vi "Confidence Interval (Power).vi"(0 "Y":dbl[](array[numeric]), 1 "confidence level":dbl=0.95, 5 "X":dbl[](array[numeric]), 7 "Weight":dbl[](array[numeric]), 9 "amplitude":dbl, 11 "power":dbl) -> (4 "Upper Bound":dbl[](array[numeric]), 6 "Lower Bound":dbl[](array[numeric]), 8 "delta amplitude":dbl, 10 "delta power":dbl, 15 "error":i32)   [LabVIEW 2020, in "NI_AALPro.lvlib"]
doc: "Calculates statistical intervals of the best power fit for a data set (<B>X</B>, <B>Y</B>). You must manually select the polymorphic instance to use."
uses:
  <vilib>/Analysis/NI_AALPro.lvlib
  <resource>/lvanlys.dll
panel:
  out "Coef. Lower Bound":dbl[](array[numeric])
  out "Coef. Upper Bound":dbl[](array[numeric])
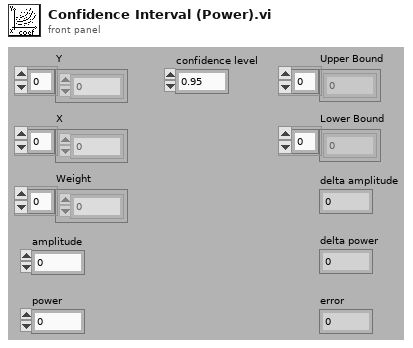
[diagram p1: front panel]
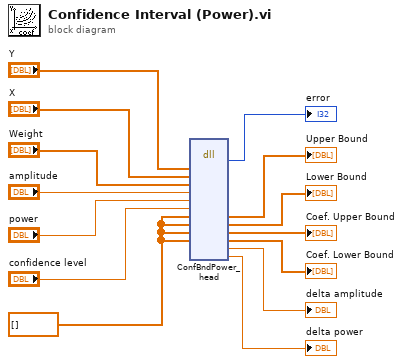
[diagram p0: block diagram]
diagram:
  w5 = dbl[] [] ("Coefficients (Upper)")
  n1 = dll-call lib="e:/builds/penguin/labview/branches/2020/dev/dist/resource/lvanlys.*" fn="ConfBndPower_head"("y"="Y", "x"="X", "weight"="Weight", "amplitude"="amplitude", "power"="power", "confidentLevel"="confidence level", "upper"=w5, "lower"=w5, "upperCoef"=w5, "lowerCoef"=w5) -> (→"error":i32, "upper"=→"Upper Bound":dbl[], "lower"=→"Lower Bound":dbl[], "upperCoef"=→"Coef. Upper Bound":dbl[], "lowerCoef"=→"Coef. Lower Bound":dbl[], "deltaAmp"=→"delta amplitude":dbl, "deltaPow"=→"delta power":dbl)  [unwired: 11 in, 2 out]
